vi "Serial Terminal Read with Echo.vi"() -> ()   [LabVIEW 2025]
doc: "This example shows how to do basic serial read communication. It also uses serial write to echo back to the terminal.s\n\nThis example expects a serial cable connected from your development PC to the RS-232 connector on the roboRIO.\n\nNote: before using this example with RS-232 you must turn off Console Out on the roboRIO. This can be done in the roboRIO Imaging Tool."
uses:
  <vilib>/Rock Robotics/WPI/SerialPort/WPI_SerialPort.ctl
panel:
  in  "Serial Port":T1
  in  "stop":bool
  out "error out":errorcluster
  out "Text Read":string
  in  "Flow Control":u16(ring) items=["None", "XON/XOFF", "RTS/CTS", "XON/XOFF & RTS/CTS", "DTR/DSR", "XON/XOFF & DTR/DSR"]
  in  "Stop Bits":u16(ring)=10 items=["1.0"=10, "1.5"=15, "2.0"=20]
  in  "Parity":u16(ring) items=["None", "Odd", "Even", "Mark", "Space"]
  in  "Data Bits":u16=8
  in  "Baud Rate":u32=115200
  # "Set these inputs before running."
  # "Controls and Input"
  # "This text is read and concatenated every 100ms"
  # "Note: before using this example you must turn off Console Out on the roboRIO.  This can be done in the roboRIO Imaging Tool"
  # "This shows wiring for serial communication.  Plug the female DB-9 connector into your PC, and then use a serial console such as PuTTY for communication testing."
  # "Female DB-9 Pinout\nfront view"
  # "DB-9\n2 (white wire)------\n3 (red wire)--------\n5 (black wire)------"
  # "roboRIO\nRS-232 TXD\nRS-232 RXD\nRS-232"
  # "5"
  # "4"
  # "3"
  # "2"
  # "1"
  # "9"
  # "8"
  # "7"
  # "6"
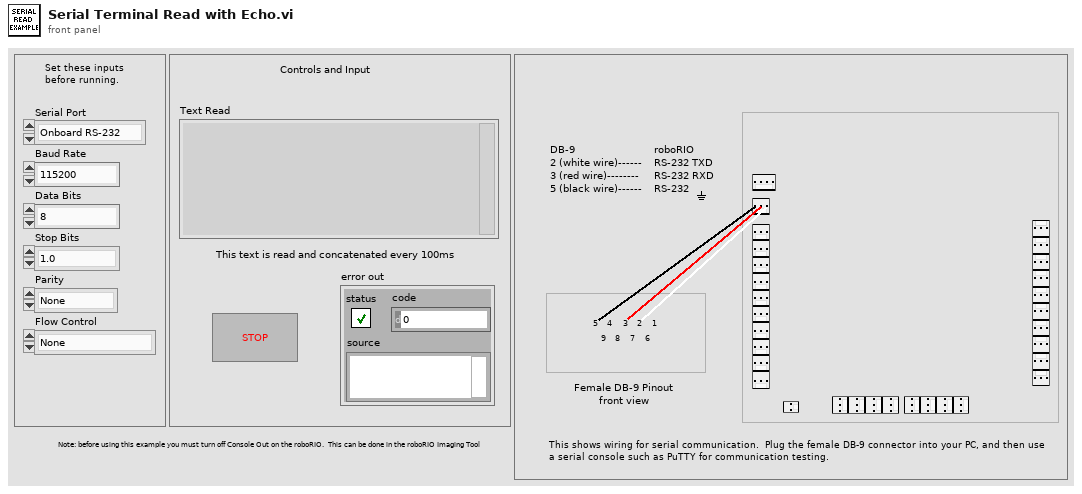
[diagram p1: front panel]
types:
  T1 = typedef "WPI_SerialPort.ctl" = enum16{"Onboard RS-232", "MXP TTL", "USB 1", "USB 2"}
  T2 = typedef "WPI_SerialPortRef.ctl" = cluster{"DevStatus":errorcluster, "Serial Port Name":refnum<visa-resource-name>}
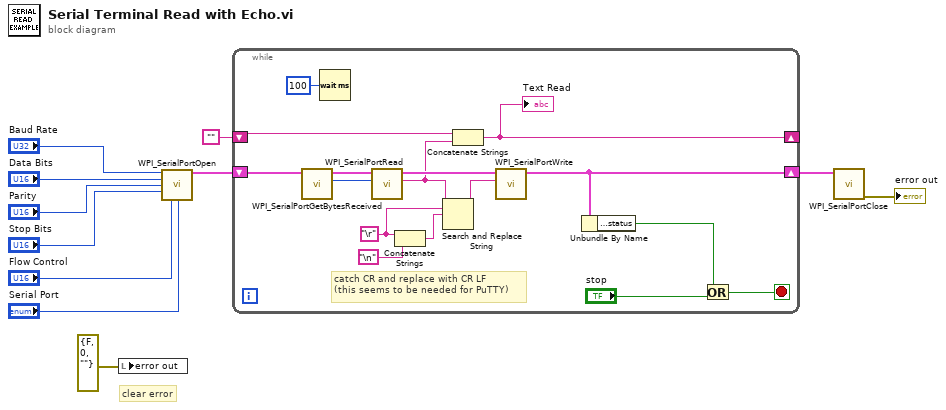
[diagram p0: block diagram]
diagram:
  # "clear error"
  n1 = local write "error out"(errorcluster {"status"=FALSE, "code"=0, "source"=""} ("error constant")) -> ()
  n2 = call <vilib>:"WPI_SerialPortOpen.vi"("Baud Rate"="Baud Rate", "Data Bits"="Data Bits", "Parity"="Parity", "Stop Bits"="Stop Bits", "Flow Control"="Flow Control", "Serial Port"="Serial Port") -> ("SerialPortRef"=w6:T2)  [unwired: 8 in, 1 out]
  n3 = while {
    shift-right: [w17] -> w5
    shift-left: w6 -> [w23]
    shift-right: [w20] -> _
    shift-left: "" -> [w19]
    stop <- w26 stop-if-true
    w12 = "\r"
    # "catch CR and replace with CR LF\n(this seems to be needed for PuTTY)"
    n4 = call <vilib>:"WPI_SerialPortGetBytesReceived.vi"("SerialPortRef"=w23) -> ("Bytes at Port"=w21:u32, "SerialPortRef"=w22:T2)  [unwired: 8 in, 1 out]
    n5 = Wait (ms)(milliseconds to wait=u32 100) -> ()  [unwired: 1 out]
    n6 = call <vilib>:"WPI_SerialPortRead.vi"("Num Bytes to Read"=w21, "SerialPortRef"=w22) -> ("Buffer"=w16:string, "SerialPortRef"=w18:T2)  [unwired: 7 in, 1 out]
    n7 = Concatenate Strings(w12, "\n") -> (w13:string)
    n8 = Search and Replace String(input string=w16, search string=w12, replace string=w13) -> (result string=w15:string)  [unwired: 5 in, 3 out]
    n9 = Concatenate Strings(w19, w16) -> (w20:string)
    "Text Read" <- w20
    n10 = call <vilib>:"WPI_SerialPortWrite.vi"("Buffer"=w15, "SerialPortRef"=w18) -> ("SerialPortRef"=w17:T2)  [unwired: 7 in, 2 out]
    n11 = Unbundle By Name(w17) -> ("DevStatus.status"=w25:bool)
    n12 = Or(x=w25, y="stop") -> (x .or. y?=w26:bool)
  }
  n13 = call <vilib>:"WPI_SerialPortClose.vi"("SerialPortRef"=w5) -> ("error out"=→"error out":errorcluster)  [unwired: 10 in]
